vi "Direct Write.vi"(8 "error in (no error)":errorcluster, 9 "Data Array":refnum<class "Generic Data.lvclass">[](array[class]), 10 "Name Array":string[](array[string]), 11 "Cluster in":refnum<class "Cluster.lvclass">) -> (0 "error out":errorcluster, 3 "Cluster out":refnum<class "Cluster.lvclass">)   [LabVIEW 2020, in "Data.lvlib" / "Cluster.lvclass"]
doc: "Write directy to the private data og the Cluster class."
uses:
  Cluster.lvclass
  Generic Data.lvclass
  Cluster.lvclass/Cluster.ctl
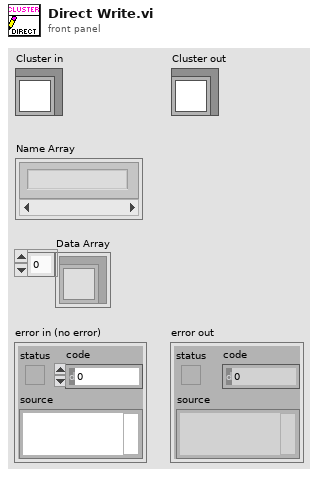
[diagram p1: front panel]
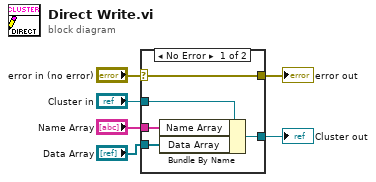
[diagram p0: block diagram]
diagram:
  n1 = case shown="No Error" "error in (no error)" {
    selector: "error in (no error)" -> [w11 w12]
    tunnel: [w11 w12] -> w5
    tunnel: [w9 w13] -> w3
    tunnel: "Cluster in" -> [w10 w13]
    tunnel: "Name Array" -> [w8 _]
    tunnel: "Data Array" -> [w7 _]
    frame No Error {
      n2 = Bundle By Name(cluster=w10, "Name Array"=w8, "Data Array"=w7) -> (w9:refnum<class "Cluster.lvclass">)
    }
    frame Error {
    }
  }
  "error out" <- w5
  "Cluster out" <- w3
